vi "Check_Ch_Name_colons.vi"(1 "No of Colons":i32, 2 "Ch Name in":string) -> (0 "Ch Name out":string)   [LabVIEW 2010]
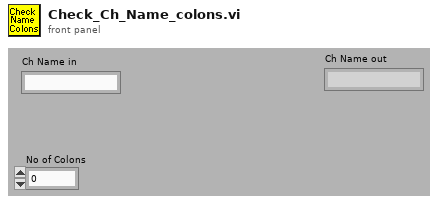
[diagram p1: front panel]
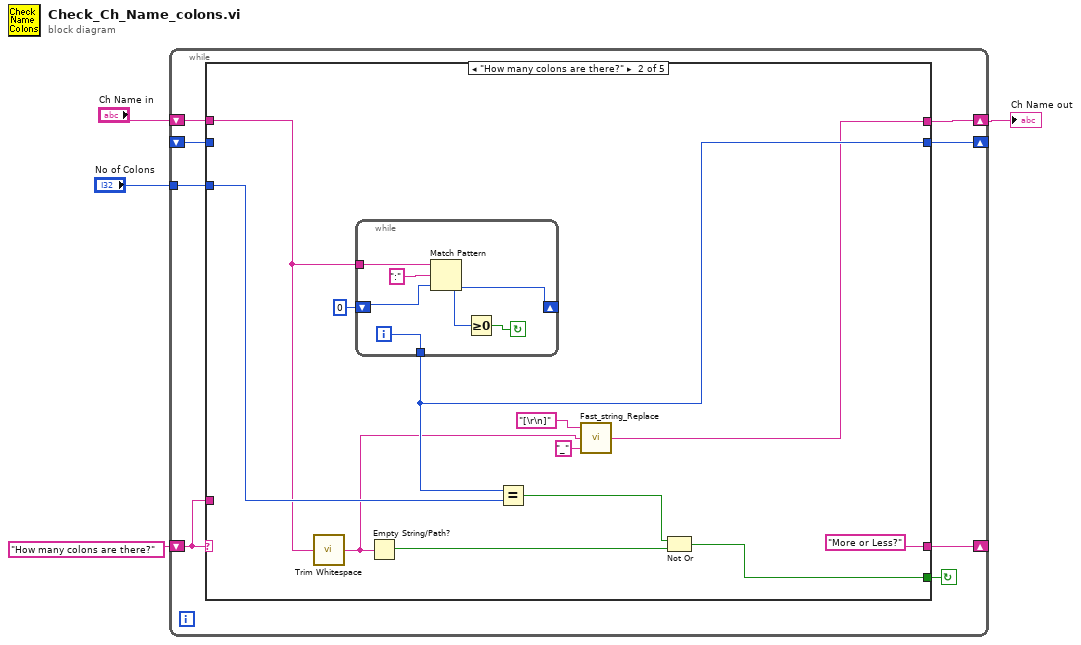
[diagram p0: block diagram]
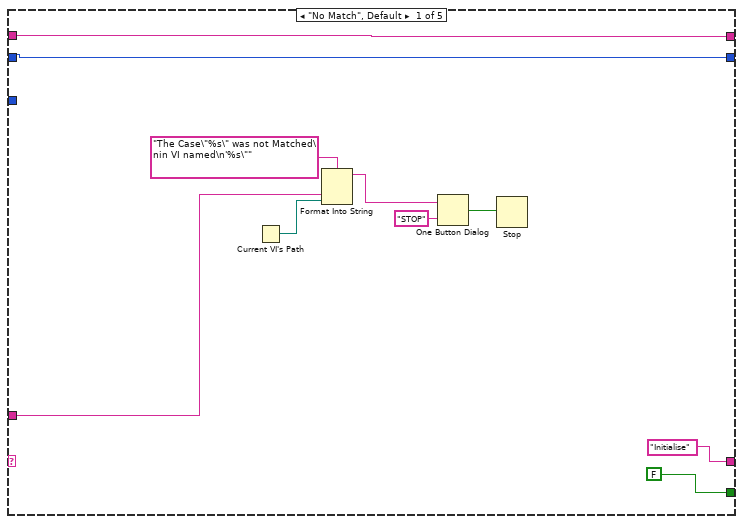
[diagram p2: hidden frame]
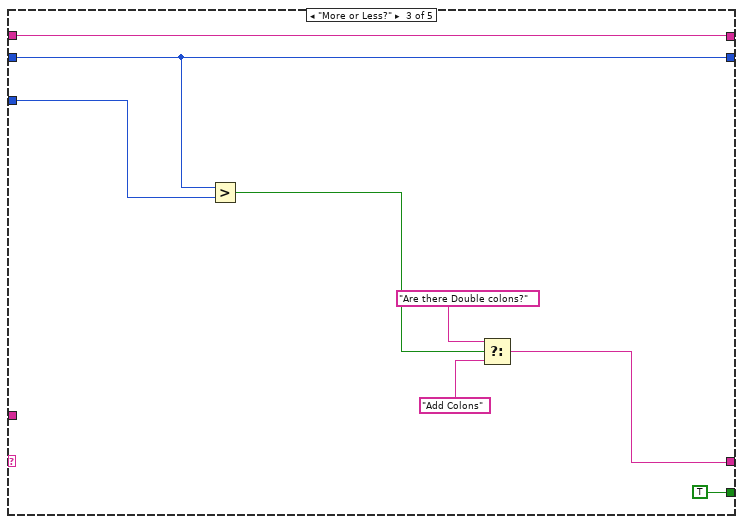
[diagram p3: hidden frame]
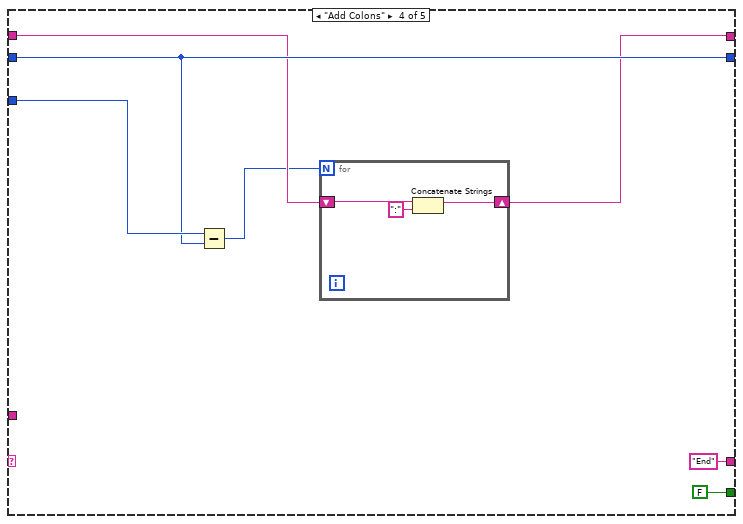
[diagram p4: hidden frame]
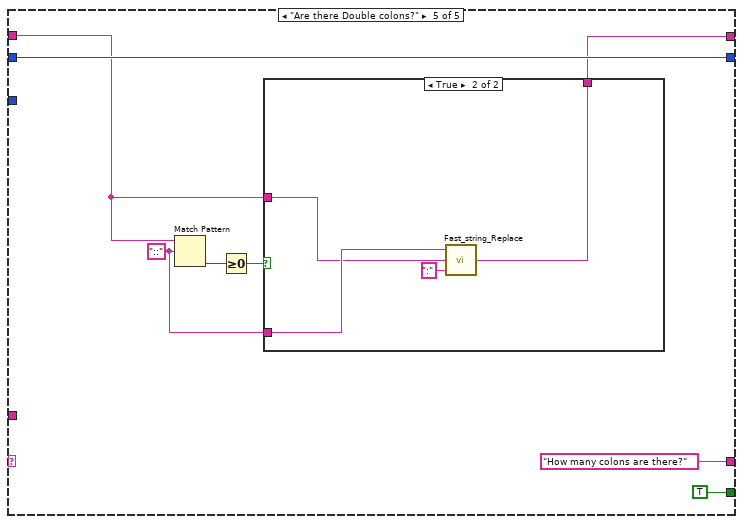
[diagram p5: hidden frame]
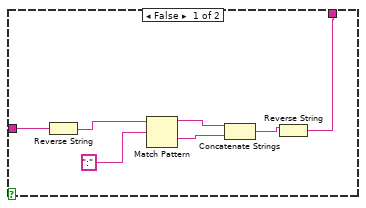
[diagram p6: hidden frame]
diagram:
  n1 = while {
    shift-left: "How many colons are there?" -> [w10]
    shift-right: [w11] -> _
    shift-right: [w8] -> w2
    shift-left: "Ch Name in" -> [w9]
    shift-right: [w7] -> _
    shift-left: _ -> [w6]
    tunnel: "No of Colons" -> [w5]
    stop <- w12 continue-if-true
    n2 = case shown="\"How many colons are there?\"" w10 {
      tunnel: [FALSE w28 TRUE FALSE TRUE] -> w12
      tunnel: ["Initialise" "More or Less?" w46 "End" "How many colons are there?"] -> w11
      tunnel: w10 -> [w17 _ _ _ _]
      tunnel: w9 -> [w14 w23 w43 w51 w60]
      tunnel: [w14 w25 w43 w52 w61] -> w8
      tunnel: w6 -> [w13 _ w42 w53 w65]
      tunnel: [w13 w32 w42 w53 w65] -> w7
      tunnel: w5 -> [_ w31 w48 w54 _]
      frame "No Match", Default {
        n3 = Current VI's Path() -> (path=w16:path)
        n4 = Format Into String(format string="The Case\"%s\" was not Matched\nin VI named\n'%s\"" ("Format String"), w17, w16) -> (resulting string=w20:string)  [unwired: 2 in, 1 out]
        n5 = One Button Dialog(message=w20, button name ("OK")="STOP") -> (true=w18:bool)
        n6 = Stop(stop? (T)=w18) -> ()
      }
      frame "How many colons are there?" {
        n7 = call <vilib>:"Trim Whitespace.vi"("string"=w23) -> ("trimmed string"=w26:string)  [unwired: 1 in]
        n8 = while {
          tunnel: w23 -> [w40]
          shift-right: [w36] -> _
          shift-left: 0 ("offset past match") -> [w38]
          tunnel: [w35] -> w32
          i -> [w35]
          stop <- w37 continue-if-true
          n9 = Match Pattern(string=w40, regular expression=":", offset (0)=w38) -> (offset past match=w36:i32)  [unwired: 3 out]
          n10 = Greater Or Equal To 0?(x=w36) -> (x >= 0?=w37:bool)
        }
        n11 = Empty String/Path?(string/path=w26) -> (empty?=w30:bool)
        n12 = Equal?(x=w32, y=w31) -> (x = y?=w29:bool)
        n13 = call "Fast_string_Replace.vi"("Replace match with:"="_", "Input String"=w26, "regular expression"="[\r\n]") -> ("Output String"=w25:string)  [unwired: 2 out]
        n14 = Not Or(1:w30, 2:w29) -> (0:w28:bool)
      }
      frame "More or Less?" {
        n15 = Greater?(x=w42, y=w48) -> (0:w47:bool)
        n16 = Select(t="Are there Double colons?", s=w47, f="Add Colons") -> (s? t:f=w46:string)
      }
      frame "Add Colons" {
        n17 = Subtract(x=w54, y=w53) -> (x-y=w50:i32)
        n18 = for {
          N: w50 -> [_]
          shift-right: [w56] -> w52
          shift-left: w51 -> [w58]
          n19 = Concatenate Strings(w58, ":" ("string")) -> (w56:string)
        }
      }
      frame "Are there Double colons?" {
        w62 = "::" ("regular expression")
        n20 = Match Pattern(string=w60, regular expression=w62) -> (offset past match=w64:i32)  [unwired: 4 out]
        n21 = Greater Or Equal To 0?(x=w64) -> (x >= 0?=w63:bool)
        n22 = case shown="True" w63 {
          tunnel: w62 -> [_ w77]
          tunnel: w60 -> [w73 w76]
          tunnel: [w67 w75] -> w61
          frame False {
            n23 = Reverse String(1:w73) -> (0:w71:string)
            n24 = Match Pattern(string=w71, regular expression=":") -> (before substring=w70:string, after substring=w69:string)  [unwired: 3 out]
            n25 = Concatenate Strings(w70, w69) -> (w68:string)
            n26 = Reverse String(1:w68) -> (0:w67:string)
          }
          frame True {
            n27 = call "Fast_string_Replace.vi"("Replace match with:"=":", "Input String"=w76, "regular expression"=w77) -> ("Output String"=w75:string)  [unwired: 2 out]
          }
        }
      }
    }
  }
  "Ch Name out" <- w2
